vi "module-07-sample-7-1-ALT.vi"() -> ()   [LabVIEW 2019]
uses:
  <vilib>/Rock Robotics/WPI/ThirdParty/JAS_Junk/TrajLib/Trajectory_Library.lvlib
  samples-common-library/Ctrl_Training_Library_Protected/CtrlTrainingLibary_Protected.lvlib
panel:
  in  "Tab Control":T1(tab)
  in  "Driver Gather Cube":bool
  in  "Driver Cancel Button":bool
  out "Request GO":bool
  out "Digital State Chart":cluster{dbl, dbl, dbl, dbl, dbl, dbl}(graph)
  out "Ready":bool
  out "Arm Extend Cmd":bool
  out "Hand Close Cmd":bool
  out "State":dbl
  out "Done Time":dbl format="%20.3f"
  out "Cur Time":dbl format="%20.3f"
  # "Training Sample 7.1 ALT\nState Machine"
  # "F1"
  # "F2"
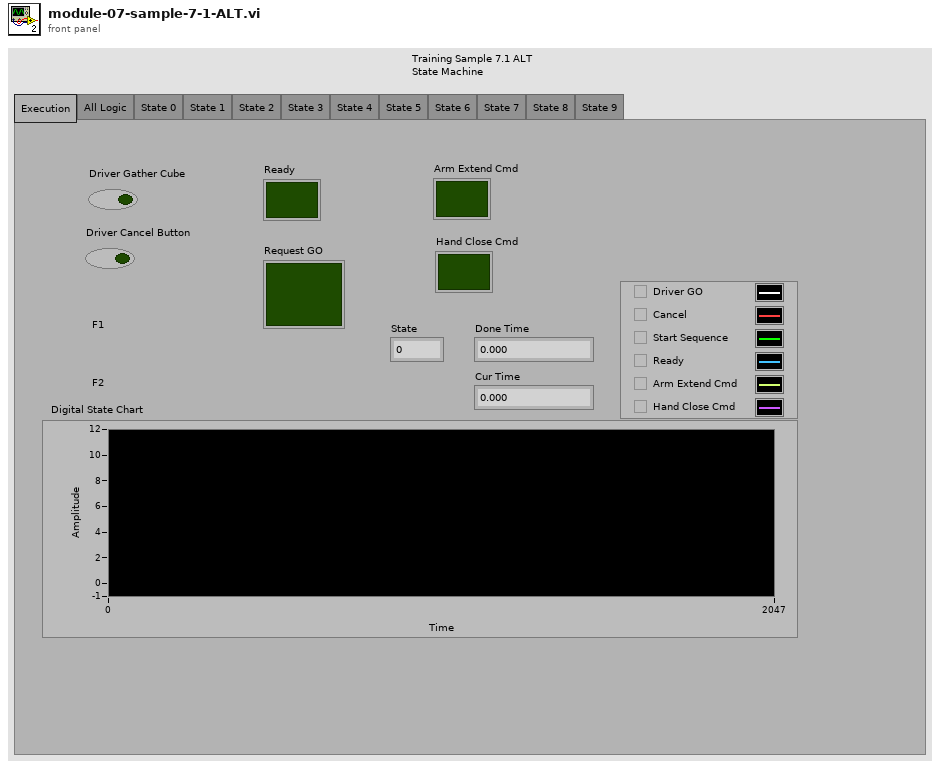
[diagram p1: front panel]
types:
  T1 = enum32{"Execution", "All Logic", "State 0", "State 1", "State 2", "State 3", "State 4", "State 5", "State 6", "State 7", "State 8", "State 9"}
  T2 = typedef "Trajectory_Library.lvlib/TIMER.ctl" = cluster{"StartTime":dbl, "Accumulated TIme":dbl, "Running":bool, "semaphore":T3}
  T3 = typedef "Semaphore RefNum" = refnum<k1>
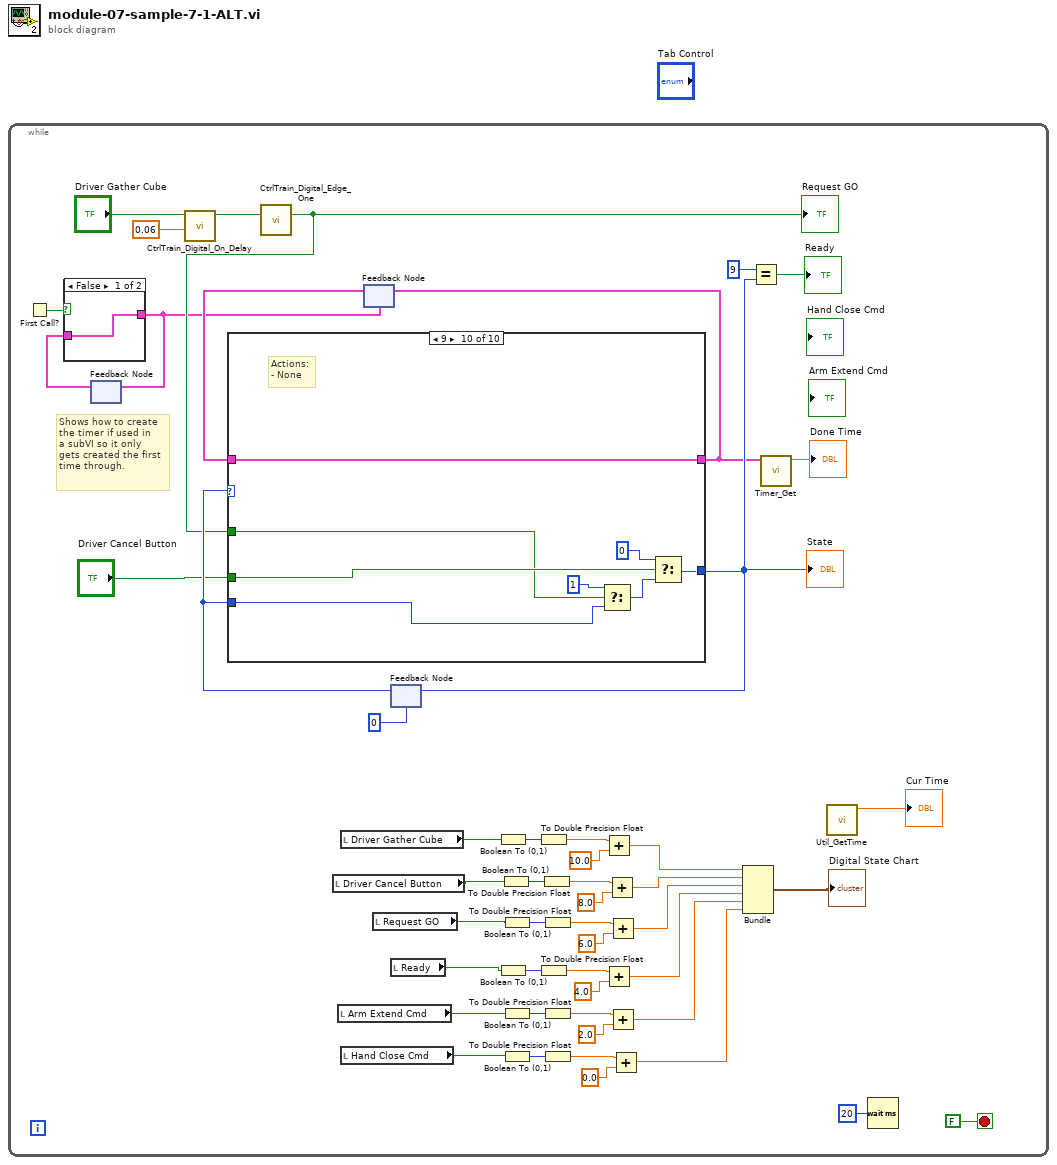
[diagram p0: block diagram]
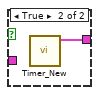
[diagram p2: hidden frame]
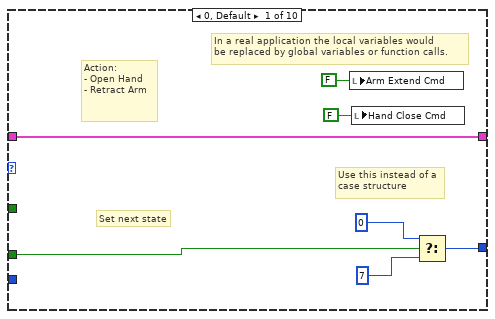
[diagram p3: hidden frame]
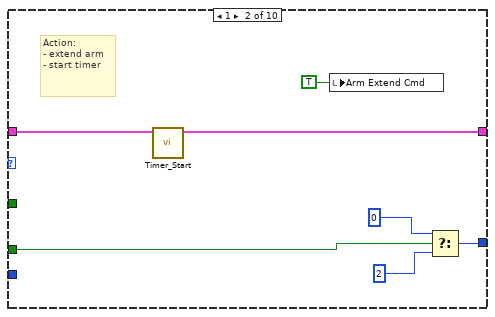
[diagram p4: hidden frame]
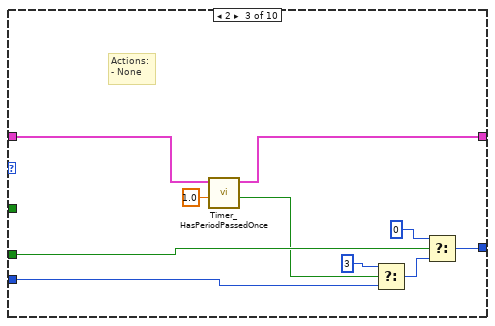
[diagram p5: hidden frame]
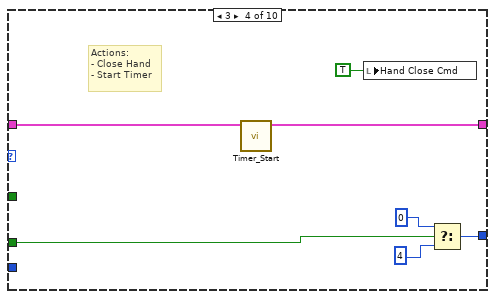
[diagram p6: hidden frame]
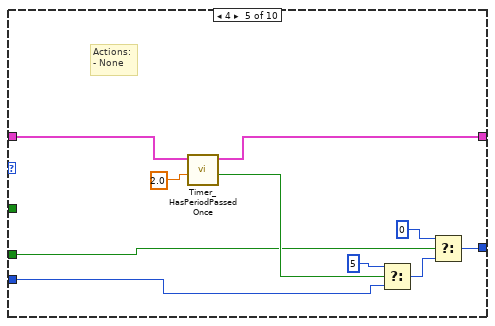
[diagram p7: hidden frame]
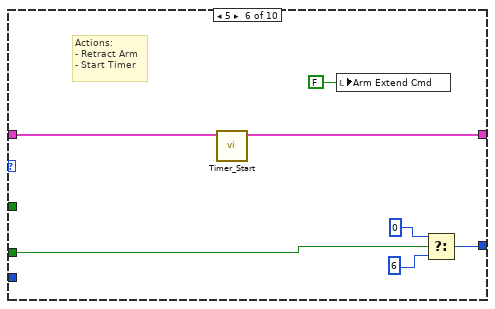
[diagram p8: hidden frame]
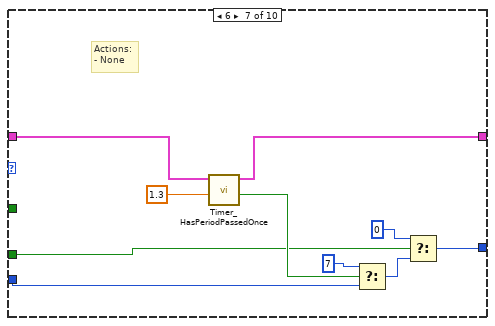
[diagram p9: hidden frame]
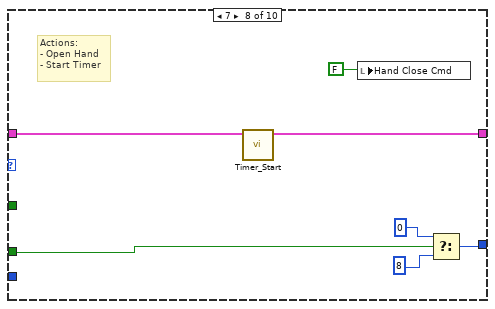
[diagram p10: hidden frame]
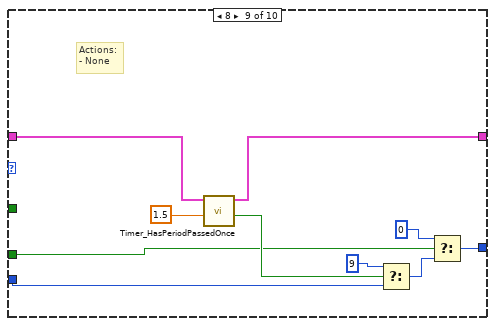
[diagram p11: hidden frame]
diagram:
  n1 = while {
    stop <- FALSE stop-if-true
    # "Shows how to create\nthe timer if used in\na subVI so it only\ngets created the first\ntime through."
    n2 = First Call?() -> (First Call?: T/F=w4:bool)
    n3 = feedback #1() -> (w2:T2)  [unwired: 1 in]
    n4 = case shown="False" w4 {
      tunnel: [w51 w52] -> w3
      tunnel: w2 -> [w51 _]
      frame False {
      }
      frame True {
        n5 = call <vilib>:"Timer_New.vi"() -> ("TIMER"=w52:T2)  [unwired: 11 in]
      }
    }
    n6 = feedback-in #1(w3) -> ()
    n7 = call "CtrlTrain_Digital_On_Delay.vi"("Delay"=0.06, "Input"="Driver Gather Cube") -> ("Output"=w14:bool)  [unwired: 8 in, 1 out]
    n8 = call "CtrlTrain_Digital_Edge_One.vi"("Input"=w14) -> ("Output"=w8:bool)  [unwired: 14 in]
    "Request GO" <- w8
    n9 = local read "Driver Cancel Button"() -> (w1:bool)
    n10 = local read "Arm Extend Cmd"() -> (w21:bool)
    n11 = local read "Driver Gather Cube"() -> (w23:bool)
    n12 = local read "Hand Close Cmd"() -> (w22:bool)
    n13 = feedback #2(w3) -> (w17:T2)
    n14 = local read "Request GO"() -> (w20:bool)
    n15 = feedback #3(u32 0) -> (w11:u32)
    n16 = case shown="9" w11 {
      tunnel: [w53 w63 w68 w78 w84 w95 w101 w112 w118 w128] -> w10
      tunnel: [w57 w60 w74 w81 w91 w99 w109 w115 w126 w135] -> w6
      tunnel: w17 -> [w57 w61 w76 w82 w92 w98 w110 w116 w127 w135]
      tunnel: w11 -> [_ _ w67 _ w87 _ w104 _ w121 w131]
      tunnel: "Driver Cancel Button" -> [w56 w62 w70 w77 w85 w94 w102 w111 w119 w130]
      tunnel: w8 -> [_ _ _ _ _ _ _ _ _ w129]
      frame 0, Default {
        # "In a real application the local variables would\nbe replaced by global variables or function calls."
        # "Use this instead of a\ncase structure"
        # "Set next state"
        # "Action:\n- Open Hand \n- Retract Arm"
        n17 = local write "Arm Extend Cmd"(FALSE ("Arm Extend Cmd")) -> ()
        n18 = local write "Hand Close Cmd"(FALSE ("Hand Close Cmd")) -> ()
        n19 = Select(t=u32 0, s=w56, f=u32 7) -> (s? t:f=w53:u32)
      }
      frame 1 {
        # "Action:\n- extend arm \n- start timer"
        n20 = call <vilib>:"Timer_Start.vi"("in Timer"=w61) -> ("out Timer"=w60:T2)  [unwired: 10 in]
        n21 = local write "Arm Extend Cmd"(TRUE ("Arm Extend Cmd")) -> ()
        n22 = Select(t=u32 0, s=w62, f=u32 2) -> (s? t:f=w63:u32)
      }
      frame 2 {
        # "Actions:\n- None"
        n23 = call <vilib>:"Timer_HasPeriodPassedOnce.vi"("Period"=1.0, "in Timer"=w76) -> ("Expired"=w69:bool, "out Timer"=w74:T2)  [unwired: 7 in, 1 out]
        n24 = Select(t=u32 3, s=w69, f=w67) -> (s? t:f=w71:u32)
        n25 = Select(t=u32 0, s=w70, f=w71) -> (s? t:f=w68:u32)
      }
      frame 3 {
        # "Actions:\n- Close Hand\n- Start Timer"
        n26 = call <vilib>:"Timer_Start.vi"("in Timer"=w82) -> ("out Timer"=w81:T2)  [unwired: 10 in]
        n27 = local write "Hand Close Cmd"(TRUE ("Hand Close Cmd")) -> ()
        n28 = Select(t=u32 0, s=w77, f=u32 4) -> (s? t:f=w78:u32)
      }
      frame 4 {
        # "Actions:\n- None"
        n29 = call <vilib>:"Timer_HasPeriodPassedOnce.vi"("Period"=2.0 ("Elapsed"), "in Timer"=w92) -> ("Expired"=w86:bool, "out Timer"=w91:T2)  [unwired: 7 in, 1 out]
        n30 = Select(t=u32 5, s=w86, f=w87) -> (s? t:f=w88:u32)
        n31 = Select(t=u32 0, s=w85, f=w88) -> (s? t:f=w84:u32)
      }
      frame 5 {
        # "Actions:\n- Retract Arm\n- Start Timer"
        n32 = call <vilib>:"Timer_Start.vi"("in Timer"=w98) -> ("out Timer"=w99:T2)  [unwired: 10 in]
        n33 = local write "Arm Extend Cmd"(FALSE ("Arm Extend Cmd")) -> ()
        n34 = Select(t=u32 0, s=w94, f=u32 6) -> (s? t:f=w95:u32)
      }
      frame 6 {
        # "Actions:\n- None"
        n35 = call <vilib>:"Timer_HasPeriodPassedOnce.vi"("Period"=1.3 ("Elapsed"), "in Timer"=w110) -> ("Expired"=w103:bool, "out Timer"=w109:T2)  [unwired: 7 in, 1 out]
        n36 = Select(t=u32 7, s=w103, f=w104) -> (s? t:f=w105:u32)
        n37 = Select(t=u32 0, s=w102, f=w105) -> (s? t:f=w101:u32)
      }
      frame 7 {
        # "Actions:\n- Open Hand\n- Start Timer"
        n38 = call <vilib>:"Timer_Start.vi"("in Timer"=w116) -> ("out Timer"=w115:T2)  [unwired: 10 in]
        n39 = local write "Hand Close Cmd"(FALSE ("Hand Close Cmd")) -> ()
        n40 = Select(t=u32 0, s=w111, f=u32 8) -> (s? t:f=w112:u32)
      }
      frame 8 {
        # "Actions:\n- None"
        n41 = call <vilib>:"Timer_HasPeriodPassedOnce.vi"("Period"=1.5 ("Elapsed"), "in Timer"=w127) -> ("Expired"=w120:bool, "out Timer"=w126:T2)  [unwired: 7 in, 1 out]
        n42 = Select(t=u32 9, s=w120, f=w121) -> (s? t:f=w122:u32)
        n43 = Select(t=u32 0, s=w119, f=w122) -> (s? t:f=w118:u32)
      }
      frame 9 {
        # "Actions:\n- None"
        n44 = Select(t=u32 1, s=w129, f=w131) -> (s? t:f=w132:u32)
        n45 = Select(t=u32 0, s=w130, f=w132) -> (s? t:f=w128:u32)
      }
    }
    "State" <- w10
    n46 = feedback-in #2(w6) -> ()
    n47 = feedback-in #3(w10) -> ()
    n48 = local read "Ready"() -> (w19:bool)
    n49 = Boolean To (0,1)(Boolean=w23) -> (0, 1=w48:i16)
    n50 = Boolean To (0,1)(Boolean=w19) -> (0, 1=w46:i16)
    n51 = Boolean To (0,1)(Boolean=w1) -> (0, 1=w43:i16)
    n52 = Boolean To (0,1)(Boolean=w20) -> (0, 1=w40:i16)
    n53 = Boolean To (0,1)(Boolean=w21) -> (0, 1=w37:i16)
    n54 = Boolean To (0,1)(Boolean=w22) -> (0, 1=w34:i16)
    n55 = To Double Precision Float(number=w48) -> (double precision float=w25:dbl)
    n56 = To Double Precision Float(number=w46) -> (double precision float=w45:dbl)
    n57 = To Double Precision Float(number=w43) -> (double precision float=w42:dbl)
    n58 = To Double Precision Float(number=w40) -> (double precision float=w39:dbl)
    n59 = To Double Precision Float(number=w37) -> (double precision float=w36:dbl)
    n60 = To Double Precision Float(number=w34) -> (double precision float=w33:dbl)
    n61 = Add(x=w25, y=10.0) -> (x+y=w24:dbl)
    n62 = Add(x=w45, y=4.0) -> (x+y=w28:dbl)
    n63 = Add(x=w42, y=8.0) -> (x+y=w30:dbl)
    n64 = Add(x=w39, y=6.0) -> (x+y=w29:dbl)
    n65 = Add(x=w36, y=2.0) -> (x+y=w32:dbl)
    n66 = Add(x=w33, y=0.0) -> (x+y=w31:dbl)
    n67 = Bundle(w24, w30, w29, w28, w32, w31) -> (→"Digital State Chart":cluster{dbl, dbl, dbl, dbl, dbl, dbl})  [unwired: 1 in]
    n68 = Equal?(x=u32 9, y=w10) -> (x = y?=→"Ready":bool)
    n69 = call <vilib>:"Timer_Get.vi"("TIMER"=w6) -> ("CurrentTImer"=→"Done Time":dbl)  [unwired: 10 in]
    n70 = call <vilib>:"Util_GetTime.vi"() -> ("FPGA_Time_Seconds"=→"Cur Time":dbl)  [unwired: 10 in, 1 out]
    n71 = Wait (ms)(milliseconds to wait=u32 20) -> ()  [unwired: 1 out]
  }
